vi "Main_PXI_v2.0.vi"() -> ()   [LabVIEW 2018]
doc: "Main VI for the controls"
uses:
  components/PMCL Dynamic Signal Analyzer/Controls/DSA excitation specs.ctl
  components/PMCL Dynamic Signal Analyzer/Controls/DSA cycle specs.ctl
  Typedefs/StateDef_Enum.ctl
  <vilib>/Utility/error.llb/DialogType.ctl
  <vilib>/Platform/TimedLoop/XDataNode/timing_clust.ctl
  <vilib>/Platform/TimedLoop/XDataNode/nitl_modes.ctl
  <vilib>/Platform/TimedLoop/XDataNode/wakeup.ctl
  <vilib>/DAQmx/read.llb/DAQmx Read (Analog 1D DBL NChan 1Samp).vi
  <vilib>/DAQmx/write.llb/DAQmx Write (Analog DBL 1Chan 1Samp).vi
  <vilib>/DAQmx/create/channels.llb/DAQmx Create Channel (AO-Voltage-Basic).vi
  <vilib>/DAQmx/create/channels.llb/DAQmx Create Channel (AI-Voltage-Basic).vi
  <vilib>/DAQmx/configure/timing.llb/DAQmx Timing (Sample Clock).vi
  <vilib>/DAQmx/create/timing.llb/DAQmx Create Timing Source (Control Loop From Task).vi
  <vilib>/DAQmx/miscellaneous.llb/DAQmx Fill In Error Info.vi
  <vilib>/Platform/TimedLoop/XDataNode/XDataNode.xnode
  Components/Timing/Timing.lvlib
  <vilib>/Platform/TimedLoop/XDataNode/XDNodeRunTimeDep.lvlib
  <vilib>/Analysis/NI_AALPro.lvlib
  <vilib>/ptbypt/NI_PtbyPt.lvlib
  <resource>/objmgr/daqmx.rc
  Components/Controller/Controller.lvlib
panel:
  in  "System Stop Button":bool
  in  "Pause chart?":bool
  in  "Controller Params":enum32{"Page 1"}(tab)
  in  "Kp":dbl=1.0 min=0.0
  in  "Controller On?":bool
  out "Status":string
  in  "Ref. Gen.":enum32{"Analog In", "Manual", "Wave Gen", "DSA"}(tab)=enum."Manual"
  in  "Ref. cmd.":dbl(slide) step=1.0 scale=-10.0..10.0 scale format="%#.1f"
  in  "Signal Cluster":T1={"phase"=0.0, "amplitude"=1.0, "frequency"=1.0, "offset"=1.0, "Signal"=enum."Square"} {"offset" format="%0.2f"; "frequency" format="%0.2f"; "amplitude" format="%0.2f"; "phase" format="%0.2f"}
  in  "Frequency\nResponse":enum16{"Plant", "RR", "CL"}(ring)
  out "DSA \nRunning?":bool
  in  "Stop \nDSA":bool
  in  "Start \nDSA":bool
  in  "DSA excitation specs":T2={"Initial Freq. [Hz]"=10.0, "Final Freq. [Hz]"=999.0, "# pts. in interval"=50, "Samping Time [s]"=0.001, "Amplitude [V]"=1.0, "Offset [V]"=0.0, "Freq Units (F: rad/s, T: Hz)"=TRUE}
  in  "Cycle Specs":T3={"Cycles To \nSettle (M)"=5, "Cycles To \nCalculate (N)"=10}
  in  "Loop Timing":enum32{"Ctrl.", "Ref. gen", "UI"}(tab)
  in  "ConvLateErrToWarning?":bool=TRUE
  in  "Ctrl.\nLoop Rate (Hz)":dbl=25000.0 format="%#_4p"
  out "# Finished\nLate counter":dbl
  out "# Finished\nLate counter":dbl
  in  "Ref. Gen.\nLoop Rate (Hz)":dbl=20000.0 format="%#_4p"
  in  "UI Loop rate (Hz)":dbl=1000.0 format="%#_6p"
  in  "Display Waveforms":enum32{"Controller Signals", "DSA "}(tab)
  out "Control Effort":dbl(graph)
  out "Waveform Chart":cluster{"Double":dbl, "Numeric":dbl}(graph)
  out "Phase Bode Plot":cluster{dbl[], dbl[]}(graph)
  out "Magnitude Bode Plot":cluster{dbl[], dbl[]}(graph)
  out "DSA Signals":cluster{"Double":dbl, "Double":dbl}(graph)
  # "Connect the Reference Signal \nto C/AI 1 of the myRIO."
  # "Pinout Config.:\nPort C/AI0 : Plant output being read           by the controller.\nPort C/AI1 : Reference signal for the control loop.\nPort C/AO0 : Control effort signal to the plant."
  # "Control Loop Timing"
  # "Ref.  Gen. Loop Timing"
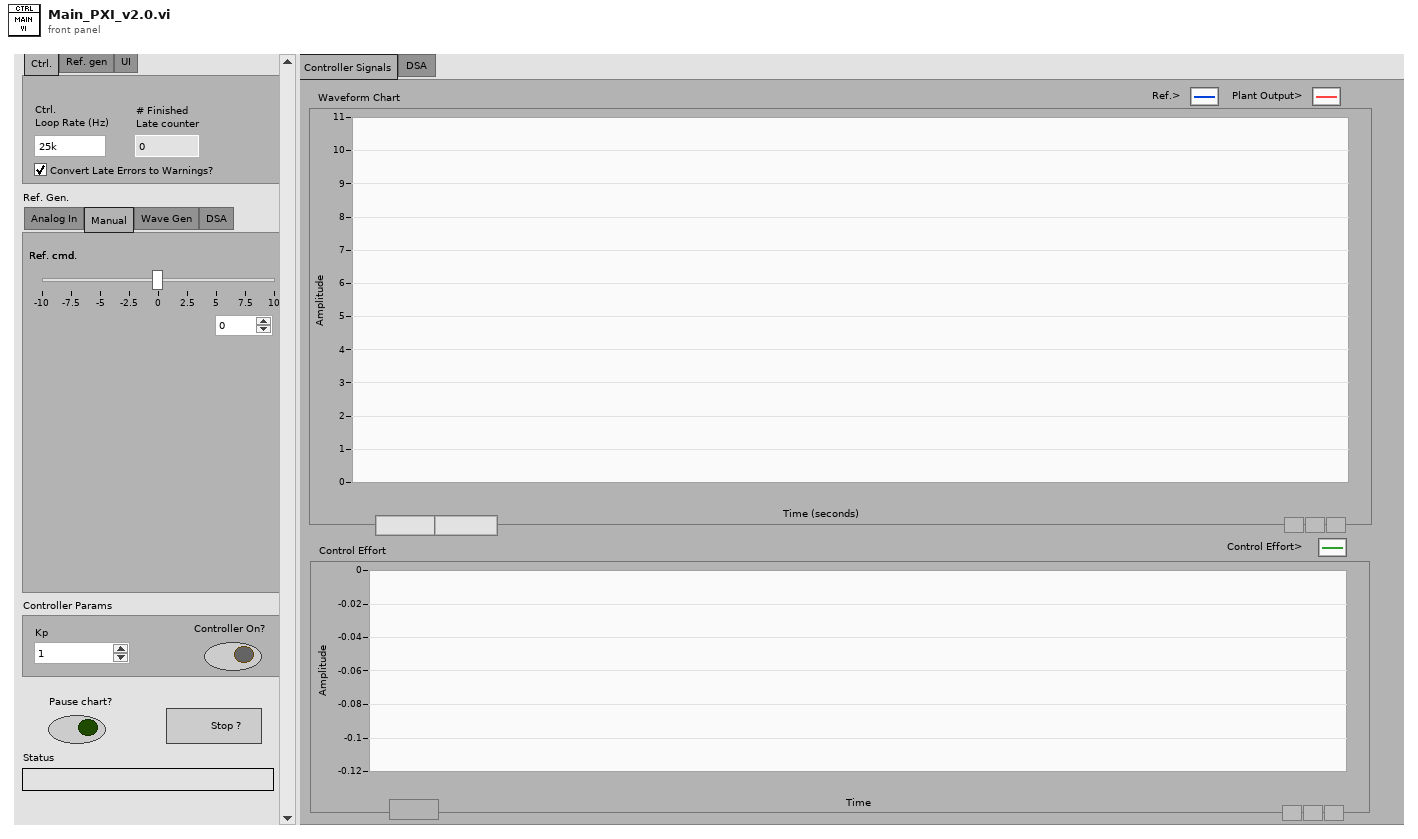
[diagram p1: front panel]
types:
  T1 = cluster{"phase":dbl, "amplitude":dbl, "frequency":dbl, "offset":dbl, "Signal":enum16{"Sine", "Square", "Sawtooth"}}
  T2 = typedef "DSA excitation specs.ctl" = cluster{"Initial Freq. [Hz]":dbl, "Final Freq. [Hz]":dbl, "# pts. in interval":i16, "Samping Time [s]":dbl, "Amplitude [V]":dbl, "Offset [V]":dbl, "Freq Units (F: rad/s, T: Hz)":bool}
  T3 = typedef "DSA cycle specs.ctl" = cluster{"Cycles To \nSettle (M)":i16, "Cycles To \nCalculate (N)":i16}
  T4 = typedef "DialogType.ctl" = u16
  T5 = typedef "StateDef_Enum.ctl" = enum16{"Initialize", "Wait", "Shutdown"}
  T6 = typedef "XDNodeRunTimeDep.lvlib/timing_clust.ctl" = cluster{"Expected End [f-1]":u64, "Actual End [f-1]":u64, "Finished Late? [f-1]":bool, "Expected End [i-1]":u64, "Actual End [i-1]":u64, "Finished Late? [i-1]":bool, "Expected Start [i]":u64, "Actual Start [i]":u64, "Expected Start [f]":u64, "Actual Start [f]":u64, "Source Name":string, "Structure Name":string, "Period":i64, "Deadline":i64, "Offset":i64, "Start":i64, "Priority":i32, "Timeout":i32, "Mode":T7, "Wakeup Reason":T8, "Error":errorcluster, "Source Type":string, "Secondary Source Type":string, "Global End Time":u64, "Global Start Time":u64, "Frame Duration":u64, "Iteration Duration":u64, "Assigned CPU":i32, "I/O Scan Engine Mode":u32}
  T7 = typedef "XDNodeRunTimeDep.lvlib/nitl_modes.ctl" = enum32{"No Change", "Process missed periods, maintain original phase", "Discard missed periods, maintain original phase", "Process missed periods, ignore original phase", "Discard missed periods, ignore original phase"}
  T8 = typedef "XDNodeRunTimeDep.lvlib/wakeup.ctl" = enum32{"Normal", "Aborted", "Asynchronous wakeup", "Timing source error", "Timed loop error", "Timeout"}
  T9 = cluster{"Analog In CH1":dbl, "Analog In CH0":dbl}
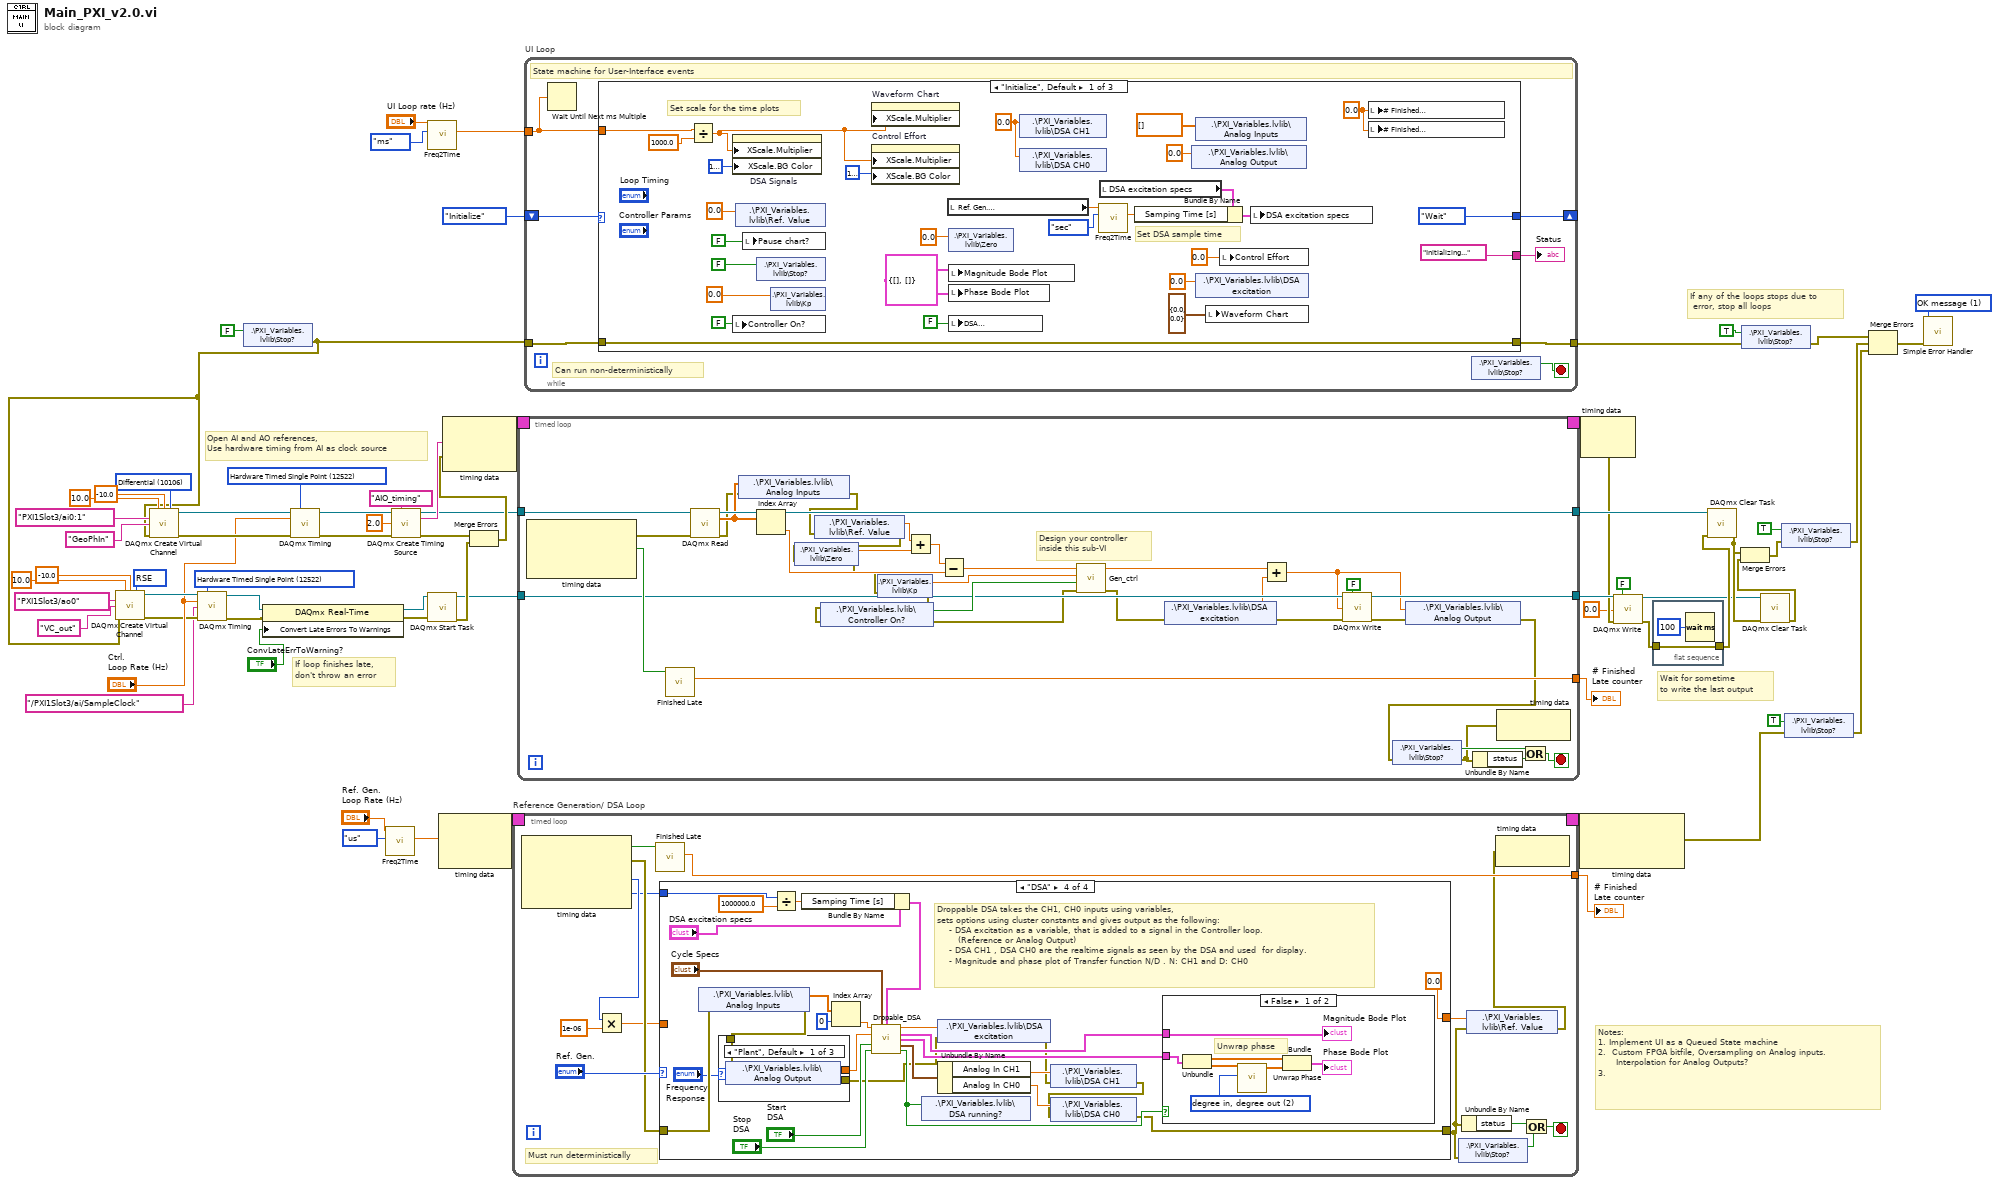
[diagram p0: block diagram]
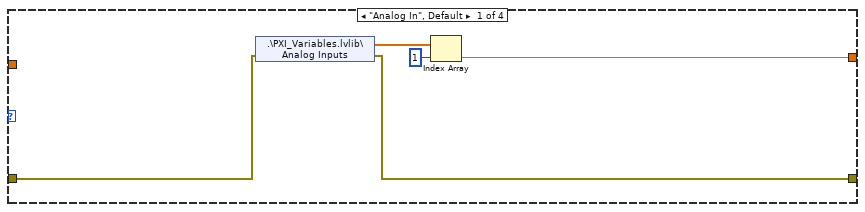
[diagram p2: hidden frame]
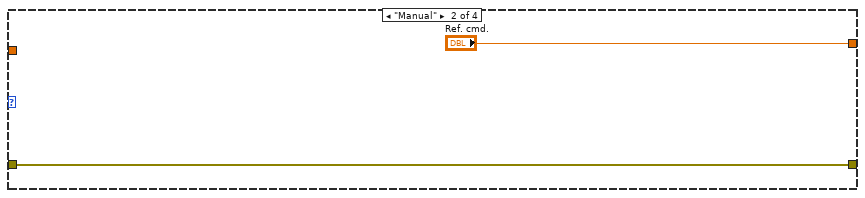
[diagram p3: hidden frame]
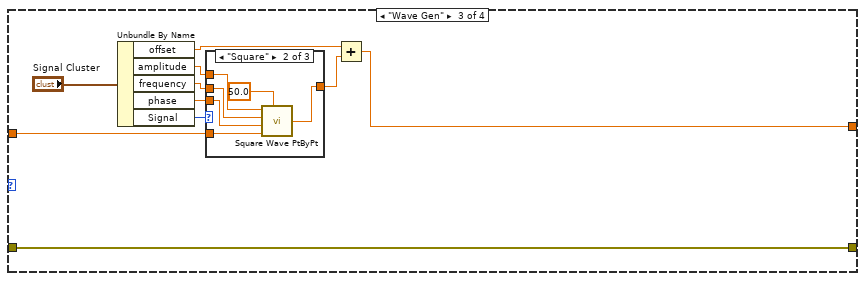
[diagram p4: hidden frame]
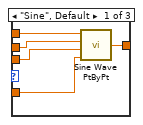
[diagram p5: hidden frame]
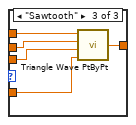
[diagram p6: hidden frame]
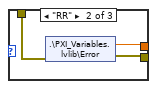
[diagram p7: hidden frame]
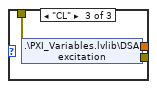
[diagram p8: hidden frame]
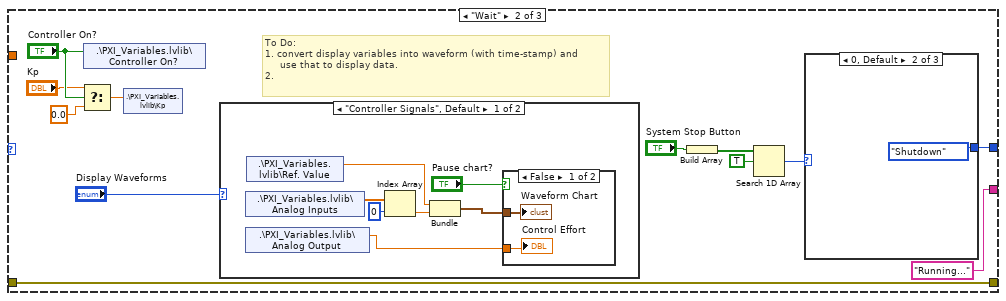
[diagram p10: hidden frame]
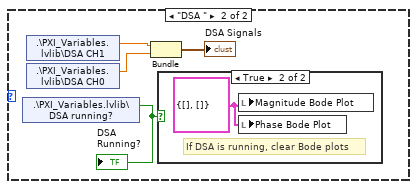
[diagram p12: hidden frame]
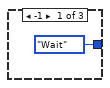
[diagram p14: hidden frame]
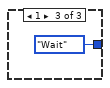
[diagram p15: hidden frame]
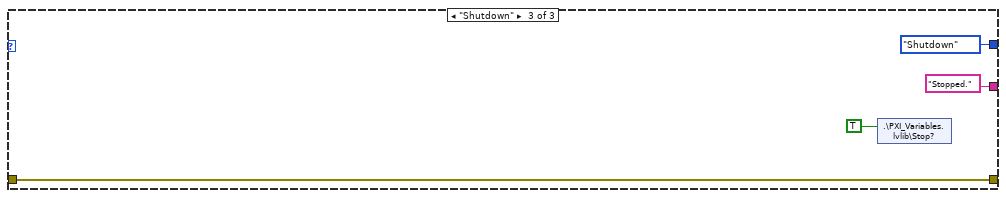
[diagram p16: hidden frame]
diagram:
  w16 = 12522 items=["Finite Samples"=10178, "Continuous Samples"=10123, "Hardware Timed Single Point"=12522] ("sample mode")
  w22 = T4 1 items=["no dialog", "OK message", "continue or stop message", "OK message + warnings", "continue/stop + warnings"] ("type of dialog (OK msg:1)")
  w31 = 12522 items=["Finite Samples"=10178, "Continuous Samples"=10123, "Hardware Timed Single Point"=12522] ("sample mode")
  w48 = 10106 items=["Default"=-1, "RSE"=10083, "NRSE"=10078, "Differential"=10106, "Pseudodifferential"=12529] ("input terminal configuration")
  w52 = 10083 items=["Default"=-1, "RSE"=10083, "Differential"=10106, "Pseudodifferential"=12529] ("output terminal configuration")
  # "Wait for sometime \nto write the last output"
  # "If loop finishes late,\ndon't throw an error"
  # "Open AI and AO references,\nUse hardware timing from AI as clock source"
  # "Notes:\n1. Implement UI as a Queued State machine\n2.  Custom FPGA bitfile, Oversampling on Analog inputs. \n      Interpolation for Analog Outputs?\n3."
  # "If any of the loops stops due to\n error, stop all loops"
  n1 = shared-variable ".\\PXI_Variables.lvlib\\Stop?"(FALSE ("Stop?")) -> (error out=w13:errorcluster)  [unwired: 1 in]
  n2 = call-poly <vilib>:"DAQmx Create Virtual Channel.vi"("maximum value"=10.0, "minimum value"=-10.0, "output terminal configuration"=w52, "physical channels"=tag "PXI1Slot3/ao0", "name to assign"="VC_out", "error in"=w13) -> ("task out"=w21:refnum<k21>, "error out"=w17:errorcluster)  [unwired: 8 in]
  n3 = call-poly <vilib>:"DAQmx Create Virtual Channel.vi"("maximum value"=10.0, "minimum value"=-10.0, "input terminal configuration"=w48, "physical channels"=tag "PXI1Slot3/ai0:1", "name to assign"="GeoPhIn", "error in"=w13) -> ("task out"=w33:refnum<k21>, "error out"=w32:errorcluster)  [unwired: 8 in]
  n4 = call-poly <vilib>:"DAQmx Timing.vi"("task/channels in"=w21, "sample mode"=w16, "rate"="Ctrl.\nLoop Rate (Hz)", "source"=tag "/PXI1Slot3/ai/SampleClock", "error in"=w17) -> ("task out"=w19:refnum<k21>, "error out"=w18:errorcluster)  [unwired: 9 in]
  n5 = property class="DAQmx Real-Time"(reference=w19, error in=w18, "Convert Late Errors To Warnings"="ConvLateErrToWarning?") -> (reference out=w24:refnum<k21>, error out=w29:errorcluster)
  n6 = call-poly <vilib>:"DAQmx Timing.vi"("task/channels in"=w33, "sample mode"=w31, "rate"="Ctrl.\nLoop Rate (Hz)", "error in"=w32) -> ("task out"=w23:refnum<k21>, "error out"=w26:errorcluster)  [unwired: 10 in]
  n7 = call "Freq2Time.vi"("Int. Time Unit"=enum16{"sec", "us", "ms"}."us", "Sample rate (Hz)"="Ref. Gen.\nLoop Rate (Hz)") -> ("Int.  time [unit]"=w12:dbl)  [unwired: 7 in, 2 out]
  n8 = call-poly <vilib>:"DAQmx Create Timing Source.vi"("task/channels in"=w23, "timing source name"="AIO_timing", "sleep time (us)"=2.0, "error in"=w26) -> ("task out"=w27:refnum<k21>, "timing source out"=w28:string, "error out"=w25:errorcluster)  [unwired: 9 in]
  n9 = call "Freq2Time.vi"("Int. Time Unit"=enum16{"sec", "us", "ms"}."ms", "Sample rate (Hz)"="UI Loop rate (Hz)") -> ("Int.  time [unit]"=w60:dbl)  [unwired: 7 in, 2 out]
  n10 = call <vilib>:"DAQmx Start Task.vi"("task/channels in"=w24, "error in"=w29) -> ("task out"=w34:refnum<k21>, "error out"=w50:errorcluster)  [unwired: 12 in]
  n11 = node-c288(w12) -> (w67:T6)  [unwired: 1 in]
  n12 = Merge Errors(w25, w50) -> (w42:errorcluster)
  n13 = node-c288(w28, w42) -> (w44:T6)
  n14 = timed-loop "Reference Generation/ DSA Loop" {
    timing: w67 -> [_]
    timing-out: [_] -> w66
    tunnel: [w82] -> w65
    stop <- w76 stop-if-true
    # "Must run deterministically"
    n15 = node-c288() -> (w83:bool, w79:errorcluster, w73:i64, w72:i64)  [unwired: 1 in]
    n16 = Multiply(x=w73, y=1e-06) -> (x*y=w75:dbl)
    n17 = call "Finished Late.vi"("Finished \nLate?"=w83) -> ("# Finished\nLate counter"=w82:dbl)  [unwired: 8 in, 2 out]
    n18 = case shown="\"DSA\"" "Ref. Gen." {
      tunnel: [w88 "Ref. cmd." w93 0.0 ("Ref. cmd.")] -> w80
      tunnel: w79 -> [w86 w89 w92 w123]
      tunnel: [w85 w89 w92 w126] -> w70
      tunnel: w75 -> [_ _ w91 _]
      tunnel: w72 -> [_ _ _ w133]
      frame "Analog In", Default {
        n19 = shared-variable ".\\PXI_Variables.lvlib\\Analog Inputs"(error in=w86) -> (w87:dbl[], error out=w85:errorcluster)
        n20 = Index Array(array=w87, index=1) -> (element=w88:dbl)
      }
      frame "Manual" {
      }
      frame "Wave Gen" {
        n21 = Unbundle By Name("Signal Cluster") -> ("offset"=w94:dbl, "amplitude"=w97:dbl, "frequency"=w96:dbl, "phase"=w95:dbl, "Signal"=w98:enum16{"Sine", "Square", "Sawtooth"})
        n22 = case shown="\"Square\"" w98 {
          tunnel: [w105 w110 w116] -> w100
          tunnel: w97 -> [w104 w109 w115]
          tunnel: w96 -> [w103 w108 w114]
          tunnel: w95 -> [w102 w107 w113]
          tunnel: w91 -> [w101 w106 w112]
          frame "Sine", Default {
            n23 = call <vilib>:"Sine Wave PtByPt.vi"("time"=w101, "phase"=w102, "frequency"=w103, "amplitude"=w104) -> ("sine wave"=w105:dbl)
          }
          frame "Square" {
            n24 = call <vilib>:"Square Wave PtByPt.vi"("amplitude"=w109, "frequency"=w108, "phase"=w107, "time"=w106, "duty cycle (%)"=50.0) -> ("square wave"=w110:dbl)
          }
          frame "Sawtooth" {
            n25 = call <vilib>:"Triangle Wave PtByPt.vi"("time"=w112, "phase"=w113, "frequency"=w114, "amplitude"=w115) -> ("triangle wave"=w116:dbl)
          }
        }
        n26 = Add(x=w94, y=w100) -> (x+y=w93:dbl)
      }
      frame "DSA" {
        # "Droppable DSA takes the CH1, CH0 inputs using variables, \nsets options using cluster constants and gives output as the following:\n    - DSA excitation as a variable, that is added to a signal in the Controller loop. \n       (Reference or Analog Output)\n    - DSA CH1 , DSA CH0 are the realtime signals as seen by the DSA and used  for display.\n    - Magnitude and phase plot of Transfer function N/D . N: CH1 and D: CH0"
        n27 = shared-variable ".\\PXI_Variables.lvlib\\Analog Inputs"(error in=w123) -> (w122:dbl[], error out=w120:errorcluster)
        n28 = case shown="\"Plant\", Default" "Frequency\nResponse" {
          tunnel: [w146 w149 w150] -> w121
          tunnel: w120 -> [w145 w147 w152]
          tunnel: [w144 w148 w151] -> w117
          frame "Plant", Default {
            n29 = shared-variable ".\\PXI_Variables.lvlib\\Analog Output"(error in=w145) -> (w146:dbl, error out=w144:errorcluster)
          }
          frame "RR" {
            n30 = shared-variable ".\\PXI_Variables.lvlib\\Error"(error in=w147) -> (w149:dbl, error out=w148:errorcluster)
          }
          frame "CL" {
            n31 = shared-variable ".\\PXI_Variables.lvlib\\DSA excitation"(error in=w152) -> (w150:dbl, error out=w151:errorcluster)
          }
        }
        n32 = Divide(x=w133, y=1000000.0) -> (x/y=w131:dbl)
        n33 = Bundle By Name(cluster="DSA excitation specs", "Samping Time [s]"=w131) -> (w130:T2)
        n34 = Index Array(array=w122, index=0) -> (element=w124:dbl)
        n35 = call "Dropable_DSA.vi"("Analog In CH1"=w124, "Cycle Specs"="Cycle Specs", "Excitation Specs"=w130, "Analog In CH0"=w121, "START"="Start \nDSA", "STOP"="Stop \nDSA") -> ("Analog Out"=w142:dbl, "Bode Magnitude"=w135:cluster{dbl[], dbl[]}, "Bode Phase"=w134:cluster{dbl[], dbl[]}, "Live signals"=w139:T9, "Running"=w129:bool)  [unwired: 4 in, 1 out]
        n36 = shared-variable ".\\PXI_Variables.lvlib\\DSA running?"(w129) -> ()  [unwired: 1 in, 1 out]
        n37 = shared-variable ".\\PXI_Variables.lvlib\\DSA excitation"(w142, error in=w117) -> (error out=w128:errorcluster)
        n38 = Unbundle By Name(w139) -> ("Analog In CH1"=w138:dbl, "Analog In CH0"=w137:dbl)
        n39 = shared-variable ".\\PXI_Variables.lvlib\\DSA CH1"(w138, error in=w128) -> (error out=w127:errorcluster)
        n40 = shared-variable ".\\PXI_Variables.lvlib\\DSA CH0"(w137, error in=w127) -> (error out=w126:errorcluster)
        n41 = case shown="False" w129 {
          tunnel: w135 -> [w153 _]
          tunnel: w134 -> [w155 _]
          frame False {
            w157 = 2 items=["radian in, radian out", "radian in, degree out", "degree in, degree out", "degree in, radian out"] ("phase unit")
            # "Unwrap phase"
            n42 = Unbundle(w155) -> (w159:dbl[], w156:dbl[])
            n43 = call <vilib>:"Unwrap Phase.vi"("phase unit"=w157, "Phase"=w156) -> ("Unwrapped Phase"=w158:dbl[])  [unwired: 8 in, 1 out]
            n44 = Bundle(w159, "Unwrapped Phase"=w158) -> (→"Phase Bode Plot":cluster{dbl[], "Unwrapped Phase":dbl[]})  [unwired: 1 in]
            "Magnitude Bode Plot" <- w153
          }
          frame True {
          }
        }
      }
    }
    n45 = shared-variable ".\\PXI_Variables.lvlib\\Stop?"(error in=w70) -> (w77:bool)  [unwired: 1 out]
    n46 = Unbundle By Name(w70) -> ("status"=w78:bool)
    n47 = shared-variable ".\\PXI_Variables.lvlib\\Ref. Value"(w80, error in=w70) -> (error out=w71:errorcluster)
    n48 = node-c288(w71) -> ()  [unwired: 1 out]
    n49 = Or(x=w78, y=w77) -> (x .or. y?=w76:bool)
  }
  "# Finished\nLate counter" <- w65
  n50 = timed-loop {
    timing: w44 -> [_]
    timing-out: [_] -> w43
    tunnel: w27 -> [w199]
    tunnel: [w197] -> w36
    tunnel: [w196] -> w35
    tunnel: w34 -> [w183]
    tunnel: [w182] -> w6
    stop <- w184 stop-if-true
    # "Design your controller \ninside this sub-VI"
    n51 = node-c288() -> (w200:errorcluster, w198:bool)  [unwired: 1 in, 1 out]
    n52 = call "Finished Late.vi"("Finished \nLate?"=w198) -> ("# Finished\nLate counter"=w197:dbl)  [unwired: 8 in, 2 out]
    n53 = call-poly <vilib>:"DAQmx Read.vi"("task/channels in"=w199, "error in"=w200) -> ("task out"=w196:refnum<k21>, "data"=w195:dbl[], "error out"=w180:errorcluster)  [unwired: 11 in]
    n54 = shared-variable ".\\PXI_Variables.lvlib\\Analog Inputs"(w195, error in=w180) -> (error out=w179:errorcluster)
    n55 = Index Array(array=w195) -> (element=w194:dbl)  [unwired: 1 in]
    n56 = shared-variable ".\\PXI_Variables.lvlib\\Ref. Value"(error in=w179) -> (w192:dbl, error out=w178:errorcluster)
    n57 = shared-variable ".\\PXI_Variables.lvlib\\Zero"(error in=w178) -> (w191:dbl, error out=w177:errorcluster)
    n58 = shared-variable ".\\PXI_Variables.lvlib\\Kp"(error in=w177) -> (w189:dbl, error out=w176:errorcluster)
    n59 = shared-variable ".\\PXI_Variables.lvlib\\Controller On?"(error in=w176) -> (w188:bool, error out=w175:errorcluster)
    n60 = Add(x=w192, y=w191) -> (x+y=w193:dbl)
    n61 = Subtract(x=w193, y=w194) -> (x-y=w190:dbl)
    n62 = call "Gen_ctrl.vi"("error in (no error)"=w175, "Controller On?"=w188, "Kp"=w189, "Error In"=w190) -> ("error out"=w174:errorcluster, "Ctrl Effort Out"=w172:dbl)  [unwired: 6 in]
    n63 = shared-variable ".\\PXI_Variables.lvlib\\DSA excitation"(error in=w174) -> (w171:dbl, error out=w173:errorcluster)
    n64 = Add(x=w172, y=w171) -> (x+y=w181:dbl)
    n65 = call-poly <vilib>:"DAQmx Write.vi"("task/channels in"=w183, "auto start"=FALSE, "data"=w181, "error in"=w173) -> ("task out"=w182:refnum<k21>, "error out"=w170:errorcluster)  [unwired: 9 in, 1 out]
    n66 = shared-variable ".\\PXI_Variables.lvlib\\Analog Output"(w181, error in=w170) -> (error out=w169:errorcluster)
    n67 = shared-variable ".\\PXI_Variables.lvlib\\Stop?"(error in=w169) -> (w187:bool, error out=w186:errorcluster)
    n68 = Unbundle By Name(w186) -> ("status"=w185:bool)
    n69 = node-c288(w186) -> ()  [unwired: 1 out]
    n70 = Or(x=w187, y=w185) -> (x .or. y?=w184:bool)
  }
  "# Finished\nLate counter" <- w36
  n71 = while "UI Loop" {
    shift-right: [w212] -> _
    shift-left: StateDef_Enum."Initialize" ("State defining Enum") -> [w213]
    tunnel: w13 -> [w211]
    tunnel: [w210] -> w59
    tunnel: w60 -> [w207]
    stop <- w208 stop-if-true
    # "Can run non-deterministically"
    # "State machine for User-Interface events"
    n72 = Wait Until Next ms Multiple(millisecond multiple=w207) -> ()  [unwired: 1 out]
    n73 = case shown="\"Initialize\", Default" w213 {
      tunnel: [StateDef_Enum."Wait" ("State defining Enum") w250 StateDef_Enum."Shutdown" ("State defining Enum")] -> w212
      tunnel: w211 -> [w238 w248 w274]
      tunnel: [w238 w248 w274] -> w210
      tunnel: ["Initializing..." ("Status") "Running..." ("Status") "Stopped." ("Status")] -> w209
      tunnel: w207 -> [w236 _ _]
      frame "Initialize", Default {
        w214 = 0.0 ("# Finished\nLate counter")
        w215 = 0.0 ("DSA CH1")
        w231 = cluster{dbl[], dbl[]} {[], []} ("Magnitude Bode Plot")
        # "Set DSA sample time"
        # "Set scale for the time plots"
        n74 = Divide(x=w236, y=1000.0) -> (x/y=w223:dbl)
        n75 = property on="DSA Signals" class="WFChart (strict)"("XScale.Multiplier"=w223, "XScale.BG Color"=u32 16777216) -> ()  [unwired: 2 in, 2 out]
        n76 = local write "Controller On?"(FALSE ("Controller On?")) -> ()
        n77 = shared-variable ".\\PXI_Variables.lvlib\\Ref. Value"(0.0 ("Ref. Value")) -> ()  [unwired: 1 in, 1 out]
        n78 = local write "Pause chart?"(FALSE ("Pause chart?")) -> ()
        n79 = shared-variable ".\\PXI_Variables.lvlib\\Stop?"(FALSE ("Stop?")) -> ()  [unwired: 1 in, 1 out]
        n80 = shared-variable ".\\PXI_Variables.lvlib\\Kp"(0.0 ("Kp")) -> ()  [unwired: 1 in, 1 out]
        n81 = property on="Waveform Chart" class="WFChart (strict)"("XScale.Multiplier"=w223) -> ()  [unwired: 2 in, 2 out]
        n82 = property on="Control Effort" class="WFChart (strict)"("XScale.Multiplier"=w223, "XScale.BG Color"=u32 16777216) -> ()  [unwired: 2 in, 2 out]
        n83 = local read "Ref. Gen.\nLoop Rate (Hz)"() -> (w226:dbl)
        n84 = shared-variable ".\\PXI_Variables.lvlib\\Zero"(0.0 ("Zero")) -> ()  [unwired: 1 in, 1 out]
        n85 = local write "Magnitude Bode Plot"(w231) -> ()
        n86 = local write "Phase Bode Plot"(w231) -> ()
        n87 = local write "DSA \nRunning?"(FALSE ("DSA \nRunning?")) -> ()
        n88 = shared-variable ".\\PXI_Variables.lvlib\\DSA CH1"(w215) -> ()  [unwired: 1 in, 1 out]
        n89 = shared-variable ".\\PXI_Variables.lvlib\\DSA CH0"(w215) -> ()  [unwired: 1 in, 1 out]
        n90 = call "Freq2Time.vi"("Int. Time Unit"=enum16{"sec", "us", "ms"}."sec", "Sample rate (Hz)"=w226) -> ("Int.  time [unit]"=w224:dbl)  [unwired: 7 in, 2 out]
        n91 = local read "DSA excitation specs"() -> (w228:T2)
        n92 = Bundle By Name(cluster=w228, "Samping Time [s]"=w224) -> (w227:T2)
        n93 = shared-variable ".\\PXI_Variables.lvlib\\Analog Output"(0.0 ("Analog Output")) -> ()  [unwired: 1 in, 1 out]
        n94 = shared-variable ".\\PXI_Variables.lvlib\\Analog Inputs"(dbl[] [] ("Analog Inputs")) -> ()  [unwired: 1 in, 1 out]
        n95 = shared-variable ".\\PXI_Variables.lvlib\\DSA excitation"(0.0 ("DSA excitation")) -> ()  [unwired: 1 in, 1 out]
        n96 = local write "Waveform Chart"(cluster{"Double":dbl, "Numeric":dbl} {"Double"=0.0, "Numeric"=0.0} ("Waveform Chart")) -> ()
        n97 = local write "Control Effort"(0.0 ("Control Effort")) -> ()
        n98 = local write "DSA excitation specs"(w227) -> ()
        n99 = local write "# Finished\nLate counter"(w214) -> ()
        n100 = local write "# Finished\nLate counter"(w214) -> ()
      }
      frame "Wait" {
        # "To Do:\n1. convert display variables into waveform (with time-stamp) and\n     use that to display data.\n2."
        n101 = Select(t="Kp", s="Controller On?", f=0.0) -> (s? t:f=w246:dbl)
        n102 = shared-variable ".\\PXI_Variables.lvlib\\Controller On?"("Controller On?") -> ()  [unwired: 1 in, 1 out]
        n103 = shared-variable ".\\PXI_Variables.lvlib\\Kp"(w246) -> ()  [unwired: 1 in, 1 out]
        n104 = case shown="\"Controller Signals\", Default" "Display Waveforms" {
          frame "Controller Signals", Default {
            n105 = shared-variable ".\\PXI_Variables.lvlib\\Analog Inputs"() -> (w260:dbl[])  [unwired: 1 in, 1 out]
            n106 = shared-variable ".\\PXI_Variables.lvlib\\Analog Output"() -> (w254:dbl)  [unwired: 1 in, 1 out]
            n107 = shared-variable ".\\PXI_Variables.lvlib\\Ref. Value"() -> (w257:dbl)  [unwired: 1 in, 1 out]
            n108 = Index Array(array=w260, index=0) -> (element=w259:dbl)
            n109 = Bundle("Double"=w257, "Numeric"=w259) -> (w255:cluster{"Double":dbl, "Numeric":dbl})  [unwired: 1 in]
            n110 = case shown="False" "Pause chart?" {
              tunnel: w255 -> [w262 _]
              tunnel: w254 -> [w261 _]
              frame False {
                "Waveform Chart" <- w262
                "Control Effort" <- w261
              }
              frame True {
              }
            }
          }
          frame "DSA " {
            n111 = shared-variable ".\\PXI_Variables.lvlib\\DSA running?"() -> (w263:bool)  [unwired: 1 in, 1 out]
            "DSA \nRunning?" <- w263
            n112 = shared-variable ".\\PXI_Variables.lvlib\\DSA CH1"() -> (w265:dbl)  [unwired: 1 in, 1 out]
            n113 = shared-variable ".\\PXI_Variables.lvlib\\DSA CH0"() -> (w264:dbl)  [unwired: 1 in, 1 out]
            n114 = Bundle("Double"=w265, "Double"=w264) -> (→"DSA Signals":cluster{"Double":dbl, "Double":dbl})  [unwired: 1 in]
            n115 = case shown="True" w263 {
              frame False {
              }
              frame True {
                w267 = cluster{dbl[], dbl[]} {[], []} ("Magnitude Bode Plot")
                # "If DSA is running, clear Bode plots"
                n116 = local write "Magnitude Bode Plot"(w267) -> ()
                n117 = local write "Phase Bode Plot"(w267) -> ()
              }
            }
          }
        }
        n118 = Build Array("System Stop Button") -> (w252:bool[])
        n119 = Search 1D Array(1D array=w252, element=TRUE) -> (index of element=w249:i32)  [unwired: 1 in]
        n120 = case shown="0, Default" w249 {
          tunnel: [StateDef_Enum."Wait" ("State defining Enum") StateDef_Enum."Shutdown" ("State defining Enum") StateDef_Enum."Wait" ("State defining Enum")] -> w250
          frame -1 {
          }
          frame 0, Default {
          }
          frame 1 {
          }
        }
      }
      frame "Shutdown" {
        n121 = shared-variable ".\\PXI_Variables.lvlib\\Stop?"(TRUE) -> ()  [unwired: 1 in, 1 out]
      }
    }
    "Status" <- w209
    n122 = shared-variable ".\\PXI_Variables.lvlib\\Stop?"() -> (w208:bool)  [unwired: 1 in, 1 out]
  }
  n123 = node-c288(w66) -> (w64:errorcluster)  [unwired: 1 out]
  n124 = node-c288(w43) -> (w5:errorcluster)
  n125 = call-poly <vilib>:"DAQmx Write.vi"("task/channels in"=w6, "auto start"=FALSE, "data"=0.0, "error in"=w5) -> ("task out"=w1:refnum<k21>, "error out"=w3:errorcluster)  [unwired: 9 in, 1 out]
  n126 = flat-sequence {
    tunnel: [w276] -> w2
    tunnel: w3 -> [w276]
    frame #0 {
      n127 = Wait (ms)(milliseconds to wait=u32 100) -> ()  [unwired: 1 out]
    }
  }
  n128 = call <vilib>:"DAQmx Clear Task.vi"("task in"=w35, "error in"=w2) -> ("error out"=w8:errorcluster)  [unwired: 13 in]
  n129 = shared-variable ".\\PXI_Variables.lvlib\\Stop?"(TRUE ("Stop?"), error in=w59) -> (error out=w58:errorcluster)
  n130 = call <vilib>:"DAQmx Clear Task.vi"("task in"=w1, "error in"=w8) -> ("error out"=w39:errorcluster)  [unwired: 13 in]
  n131 = Merge Errors(w8, w39) -> (w40:errorcluster)
  n132 = shared-variable ".\\PXI_Variables.lvlib\\Stop?"(TRUE ("Stop?"), error in=w40) -> (error out=w37:errorcluster)
  n133 = shared-variable ".\\PXI_Variables.lvlib\\Stop?"(TRUE ("Stop?"), error in=w64) -> (error out=w38:errorcluster)
  n134 = Merge Errors(w58, w37, w38) -> (w68:errorcluster)
  n135 = call <vilib>:"Simple Error Handler.vi"("type of dialog (OK msg:1)"=w22, "error in (no error)"=w68) -> ()  [unwired: 3 in, 5 out]
